vi "GenerateINIPath.vi"() -> (3 "INI Path":path)   [LabVIEW 2017, in "Client.lvlib"]
uses:
  Client.lvlib
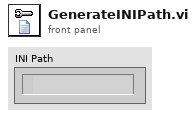
[diagram p1: front panel]
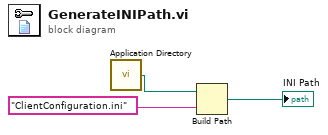
[diagram p0: block diagram]
diagram:
  n1 = call <vilib>:"Application Directory.vi"() -> ("Application Directory"=w1:path)
  n2 = Build Path(base path=w1, name or relative path="ClientConfiguration.ini") -> (appended path=→"INI Path":path)
